vi "sub_ledmatrix_data-to-arduino.vi"(8 "error in":errorcluster) -> (0 "error out":errorcluster, 3 "data out":string)   [LabVIEW 2019]
uses:
  Ctrl/cmd_common.ctl
  Ctrl/joystick_opval.ctl
panel:
  in  "index":u8
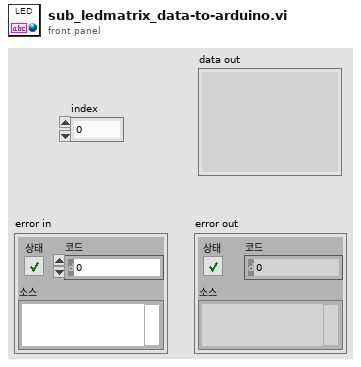
[diagram p1: front panel]
types:
  T1 = typedef "cmd_common.ctl" = enum16{"read", "write"}
  T2 = typedef "joystick_opval.ctl" = cluster{"curr":u32, "last":u32}
  T3 = typedef "ledmatrix_data.ctl" = cluster{"ip":string, "data":string, "Port":refnum<visa-resource-name>, "time":string}
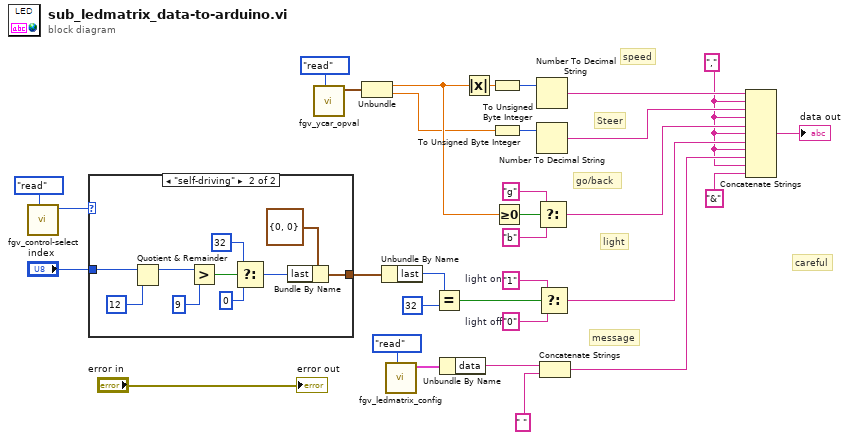
[diagram p0: block diagram]
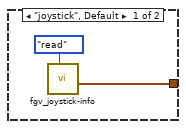
[diagram p2: hidden frame]
diagram:
  w23 = "0"  # light off
  w22 = "1"  # light on
  w18 = "," ("string")
  # "careful"
  # "message"
  # "light"
  # "go/back"
  # "Steer"
  # "speed"
  n1 = call "fgv_control-select.vi"("cmd"=cmd_common."read") -> ("mode out"=w10:enum16{"joystick", "self-driving"})  [unwired: 10 in]
  n2 = case shown="\"self-driving\"" w10 {
    tunnel: [w34 w43] -> w8
    tunnel: "index" -> [_ w37]
    frame "joystick", Default {
      n3 = call "fgv_joystick-info.vi"("init"=enum16{"enable", "init", "read", "write"}."read") -> ("opval"=w34:T2)  [unwired: 7 in, 3 out]
    }
    frame "self-driving" {
      n4 = Quotient & Remainder(x=w37, y=u8 12) -> (x-y*floor(x/y)=w35:u8)  [unwired: 1 out]
      n5 = Greater?(x=w35, y=u8 9) -> (0:w41:bool)
      n6 = Select(t=u8 32 ("y"), s=w41, f=u8 0 ("y")) -> (s? t:f=w42:u8)
      n7 = Bundle By Name(cluster=T2 {"curr"=0, "last"=0} ("opval"), "last"=w42) -> (w43:T2)
    }
  }
  n8 = call "fgv_ycar_opval.vi"("cmd"=enum16{"read", "write", "ini"}."read") -> ("opval out"=w4:cluster{"speed":dbl, "steer":dbl})  [unwired: 10 in]
  n9 = Unbundle(w4) -> ("speed"=w7:dbl, "steer"=w6:dbl)
  n10 = Unbundle By Name(w8) -> ("last"=w30:u32)
  n11 = call "fgv_ledmatrix_config.vi"("cmd"=cmd_common."read") -> ("data out"=w2:T3)  [unwired: 10 in]
  n12 = Equal?(x=w30, y=u32 32) -> (x = y?=w31:bool)
  n13 = Unbundle By Name(w2) -> ("data"=w1:string)
  n14 = Absolute Value(x=w7) -> (abs(x)=w13:dbl)
  n15 = To Unsigned Byte Integer(number=w13) -> (unsigned 8bit integer=w11:u8)
  n16 = To Unsigned Byte Integer(number=w6) -> (unsigned 8bit integer=w12:u8)
  n17 = Greater Or Equal To 0?(x=w7) -> (x >= 0?=w27:bool)
  n18 = Number To Decimal String(number=w11) -> (decimal integer string=w25:string)  [unwired: 1 in]
  n19 = Number To Decimal String(number=w12) -> (decimal integer string=w26:string)  [unwired: 1 in]
  n20 = Select(t="g" ("string"), s=w27, f="b" ("string")) -> (s? t:f=w28:string)
  n21 = Select(t=w22, s=w31, f=w23) -> (s? t:f=w29:string)
  n22 = Concatenate Strings(w1, " " ("문자열")) -> (w32:string)
  n23 = Concatenate Strings(w25, w18, w26, w18, w28, w18, w29, w18, w32, w18, "&" ("string")) -> (→"data out":string)
  "error out" <- "error in"
